vi "Generate noise.vi"(6 "noisehifreq":dbl, 9 "noise std":dbl, 10 "input dt":dbl, 11 "samples":i32) -> (2 "noise deriv":dbl[](array[numeric]), 3 "noise":dbl[](array[numeric]))   [LabVIEW 2012]
uses:
  <vilib>/Analysis/3filter.llb/Filter Passband Type.ctl
  <vilib>/Analysis/3filter.llb/Butterworth Filter (DBL).vi
  <vilib>/Analysis/NI_AALBase.lvlib
  <vilib>/Analysis/NI_AALPro.lvlib
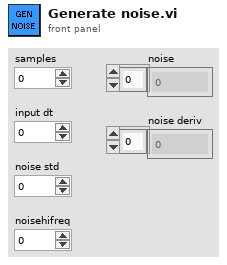
[diagram p1: front panel]
types:
  T1 = typedef "NI_AALBase.lvlib/Filter Passband Type.ctl" = enum32{"Lowpass", "Highpass", "Bandpass", "Bandstop"}
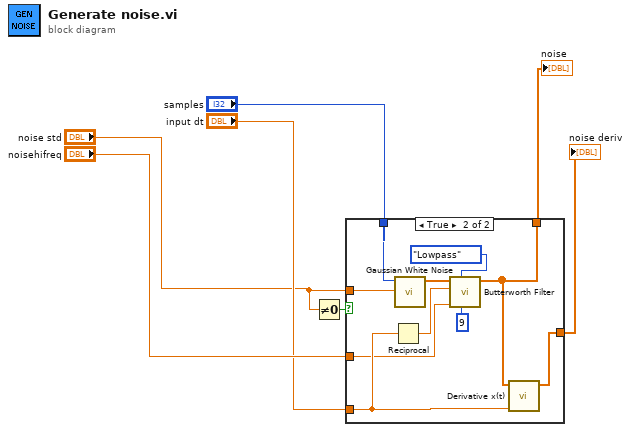
[diagram p0: block diagram]
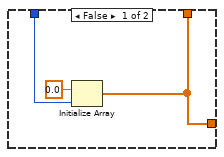
[diagram p2: hidden frame]
diagram:
  n1 = Not Equal To 0?(x="noise std") -> (x != 0?=w4:bool)
  n2 = case shown="True" w4 {
    tunnel: "noise std" -> [_ w20]
    tunnel: "samples" -> [w10 w19]
    tunnel: "input dt" -> [_ w16]
    tunnel: [w8 w12] -> w5
    tunnel: [w8 w18] -> w6
    tunnel: "noisehifreq" -> [_ w11]
    frame False {
      n3 = Initialize Array(0.0 ("element"), w10) -> (w8:dbl[])
    }
    frame True {
      n4 = Reciprocal(x=w16) -> (1/x=w15:dbl)
      n5 = call <vilib>:"Gaussian White Noise.vi"("standard deviation"=w20, "samples"=w19) -> ("Gaussian noise pattern"=w17:dbl[])  [unwired: 8 in, 1 out]
      n6 = call-poly <vilib>:"Butterworth Filter.vi"("order"=9, "filter type"=Filter_Passband_Type."Lowpass", "low cutoff freq: fl"=w11, "sampling freq: fs"=w15, "X"=w17) -> ("Filtered X"=w12:dbl[])  [unwired: 3 in, 1 out]
      n7 = call <vilib>:"Derivative x(t).vi"("dt"=w16, "X"=w12) -> ("dX/dt"=w18:dbl[])  [unwired: 8 in, 1 out]
    }
  }
  "noise deriv" <- w6
  "noise" <- w5
